vi "maze_v7.vi"   [LabVIEW 2012]
uses:
  <vilib>/NXT/Subs/MotorOutput.ctl
  <vilib>/NXT/Block Support/NXT_InputPort.ctl
  <vilib>/NXT/Dual Mode Library/Motors/MotorBrake.vi
  <vilib>/NXT/Dual Mode Library/Motors/MotorOn.vi
  <vilib>/NXT/Dual Mode Library/Motors/MotorReverse.vi
  <vilib>/NXT/Dual Mode Library/prims/addArrayElements_int.vi
  <vilib>/NXT/Dual Mode Library/Waits/Wait_Num(msec).vi
  <vilib>/NXT/Dual Mode Library/Sound/Tone.vi
types:
  T1 = typedef "MotorOutput.ctl" = u8
  T2 = typedef "LVHSConnector.ctl" = cluster{"Hardware":string, "Flattened String":string}
  T3 = typedef "NXT_InputPort.ctl" = u8
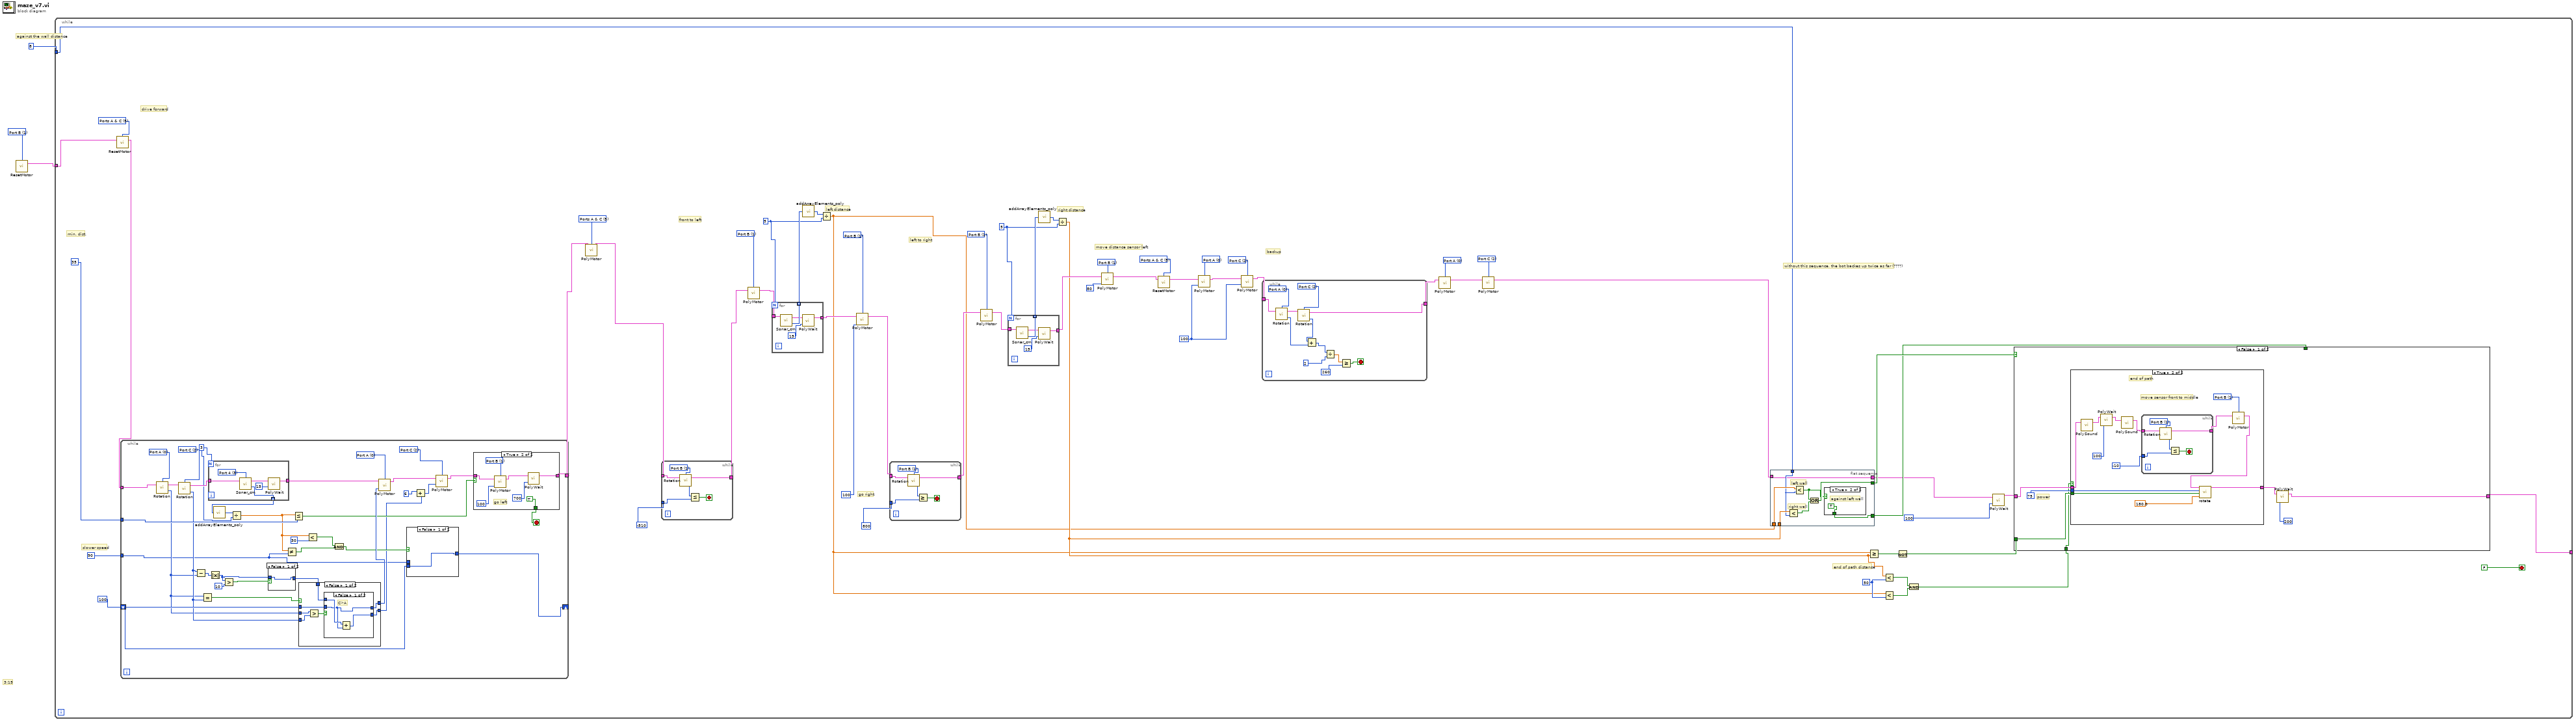
[diagram p0: block diagram]
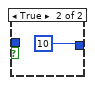
[diagram p2: hidden frame]
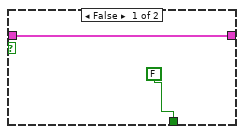
[diagram p4: hidden frame]
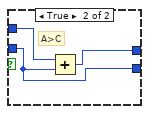
[diagram p5: hidden frame]
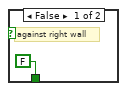
[diagram p7: hidden frame]
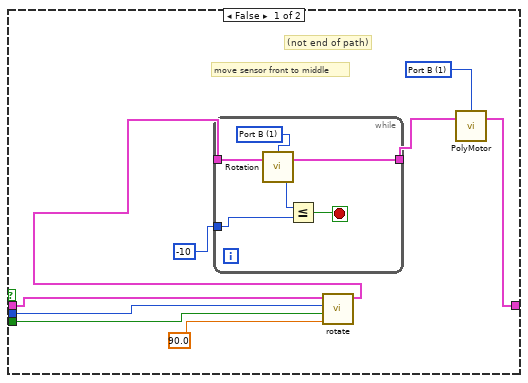
[diagram p8: hidden frame]
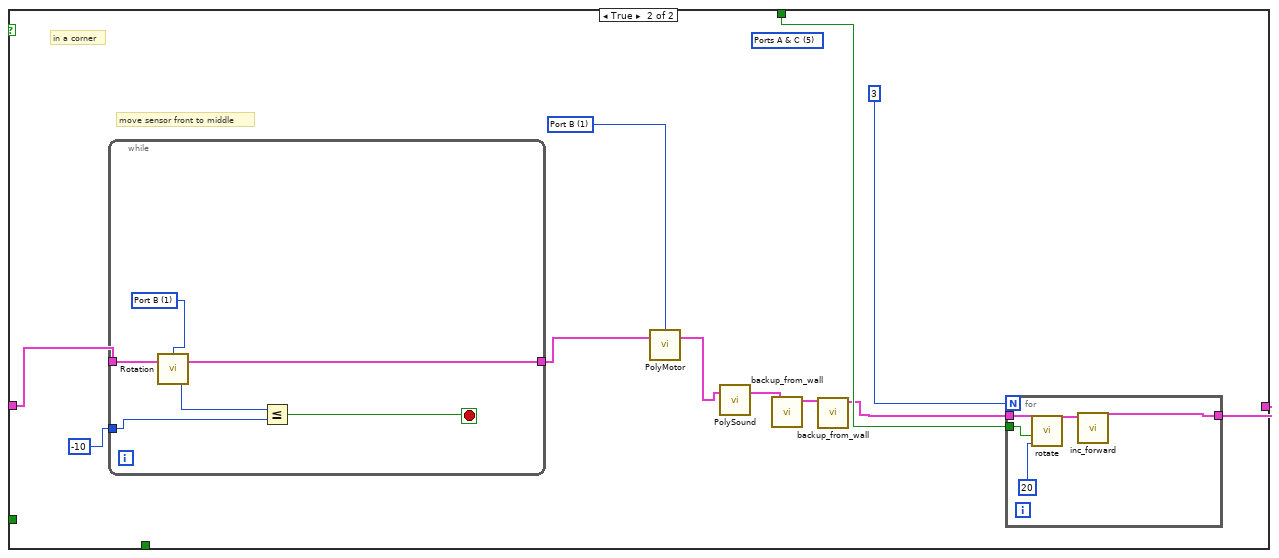
[diagram p9: hidden frame]
diagram:
  w3 = T1 1 items=["Port A"=0, "Port B"=1, "Port C"=2, "Ports A & B"=4, "Ports A & C"=5, "Ports B & C"=6, "All Ports"=3] ("Output Port (All Ports)")
  # "3:15"
  # "against the wall distance"
  n1 = call <vilib>:"ResetMotor.vi"("Port (All Ports)"=w3) -> ("NXT"=w1:T2)  [unwired: 3 in]
  n2 = while {
    tunnel: u16 8 ("power") -> [w57]
    tunnel: [w54] -> _
    tunnel: w1 -> [w46]
    stop <- FALSE stop-if-true
    w7 = u16 50 ("power")
    w14 = T1 1 items=["Port A"=0, "Port B"=1, "Port C"=2, "Ports A & B"=4, "Ports A & C"=5, "Ports B & C"=6, "All Ports"=3] ("Output Port (All Ports)")
    w19 = T1 2 items=["Port A"=0, "Port B"=1, "Port C"=2, "Ports A & B"=4, "Ports A & C"=5, "Ports B & C"=6, "All Ports"=3] ("Output Port (All Ports)")
    w17 = T1 0 items=["Port A"=0, "Port B"=1, "Port C"=2, "Ports A & B"=4, "Ports A & C"=5, "Ports B & C"=6, "All Ports"=3] ("Output Port (All Ports)")
    w21 = 100
    w23 = T1 2 items=["Port A"=0, "Port B"=1, "Port C"=2, "Ports A & B"=4, "Ports A & C"=5, "Ports B & C"=6, "All Ports"=3] ("Output Port (All Ports)")
    w25 = T1 0 items=["Port A"=0, "Port B"=1, "Port C"=2, "Ports A & B"=4, "Ports A & C"=5, "Ports B & C"=6, "All Ports"=3] ("Output Port (All Ports)")
    w26 = T1 5 items=["Port A"=0, "Port B"=1, "Port C"=2, "Ports A & B"=4, "Ports A & C"=5, "Ports B & C"=6, "All Ports"=3] ("Output Port (All Ports)")
    w29 = 5
    w32 = 5
    w39 = T1 1 items=["Port A"=0, "Port B"=1, "Port C"=2, "Ports A & B"=4, "Ports A & C"=5, "Ports B & C"=6, "All Ports"=3] ("Output Port (All Ports)")
    w40 = T1 1 items=["Port A"=0, "Port B"=1, "Port C"=2, "Ports A & B"=4, "Ports A & C"=5, "Ports B & C"=6, "All Ports"=3] ("Output Port (All Ports)")
    w44 = T1 1 items=["Port A"=0, "Port B"=1, "Port C"=2, "Ports A & B"=4, "Ports A & C"=5, "Ports B & C"=6, "All Ports"=3] ("Output Port (All Ports)")
    w53 = T1 5 items=["Port A"=0, "Port B"=1, "Port C"=2, "Ports A & B"=4, "Ports A & C"=5, "Ports B & C"=6, "All Ports"=3] ("Output Port (All Ports)")
    w51 = T1 5 items=["Port A"=0, "Port B"=1, "Port C"=2, "Ports A & B"=4, "Ports A & C"=5, "Ports B & C"=6, "All Ports"=3] ("Output Port (All Ports)")
    # "end of path distance"
    # "move distance sensor left"
    # "backup"
    # "right distance"
    # "left distance"
    # "go right"
    # "left to right"
    # "front to left"
    # "drive forward"
    # "min. dist."
    # "slower speed"
    # "without this sequence, the bot backes up twice as far (????)"
    n3 = call <vilib>:"ResetMotor.vi"("NXT"=w46, "Port (All Ports)"=w51) -> ("NXT"=w52:T2)  [unwired: 2 in]
    n4 = while {
      tunnel: w52 -> [w133]
      tunnel: [w121] -> w50
      tunnel: 35 -> [w123]
      shift-right: [w113] -> _
      shift-left: 100 -> [w112]
      tunnel: 90 -> [w97]
      stop <- w118 stop-if-true
      w98 = 3
      w126 = T1 2 items=["Port A"=0, "Port B"=1, "Port C"=2, "Ports A & B"=4, "Ports A & C"=5, "Ports B & C"=6, "All Ports"=3] ("Output Port (All Ports)")
      w127 = T1 0 items=["Port A"=0, "Port B"=1, "Port C"=2, "Ports A & B"=4, "Ports A & C"=5, "Ports B & C"=6, "All Ports"=3] ("Output Port (All Ports)")
      w128 = T1 2 items=["Port A"=0, "Port B"=1, "Port C"=2, "Ports A & B"=4, "Ports A & C"=5, "Ports B & C"=6, "All Ports"=3] ("Output Port (All Ports)")
      w129 = T1 0 items=["Port A"=0, "Port B"=1, "Port C"=2, "Ports A & B"=4, "Ports A & C"=5, "Ports B & C"=6, "All Ports"=3] ("Output Port (All Ports)")
      n5 = call <vilib>:"Rotation.vi"("NXT"=w133, "Port (Port A)"=w127) -> ("Angle of Rotation"=w110:i32, "NXT"=w132:T2)  [unwired: 1 in]
      n6 = call <vilib>:"Rotation.vi"("NXT"=w132, "Port (Port A)"=w126) -> ("Angle of Rotation"=w111:i32, "NXT"=w131:T2)  [unwired: 1 in]
      n7 = Subtract(x=w111, y=w110) -> (x-y=w109:i32)
      n8 = Equal?(x=w110, y=w111) -> (x = y?=w125:bool)
      n9 = for {
        N: w98 -> [_]
        tunnel: w131 -> [w138]
        tunnel: [w136] -> w124
        tunnel: [w137] -> w101 mode=indexing
        w139 = T3 3 items=["Port 1", "Port 2", "Port 3", "Port 4"] ("Port (Port 4)")
        n10 = call <vilib>:"Sonar_cm.vi"("NXT"=w138, "Port (Port 4)"=w139) -> ("Distance (cm)"=w137:i16, "NXT"=w135:T2)  [unwired: 1 in]
        n11 = call-poly <vilib>:"PolyWait.vi"("Time (100 msec)"=15, "NXT"=w135) -> ("NXT"=w136:T2)  [unwired: 2 in]
      }
      n12 = Absolute Value(x=w109) -> (abs(x)=w106:i32)
      n13 = call-poly <vilib>:"addArrayElements_poly.vi"("Numeric Array"=w101) -> ("Sum"=w100:i32)
      n14 = Greater?(x=w106, y=10) -> (0:w107:bool)
      n15 = Divide(x=w100, y=w98) -> (x/y=w99:dbl)
      n16 = case shown="False" w107 {
        tunnel: [w140 10] -> w105
        tunnel: w106 -> [w140 _]
        frame False {
        }
        frame True {
        }
      }
      n17 = Not Equal?(x=w99, y=w97) -> (x != y?=w115:bool)
      n18 = Less Or Equal?(x=w99, y=w123) -> (x <= y?=w119:bool)
      n19 = case shown="False" w125 {
        tunnel: [w157 w166] -> w122
        tunnel: w112 -> [w158 w166]
        tunnel: [w156 w166] -> w103
        tunnel: w111 -> [w155 _]
        tunnel: w110 -> [w154 _]
        tunnel: w105 -> [w153 _]
        frame False {
          n20 = Greater?(x=w154, y=w155) -> (0:w159:bool)
          n21 = case shown="False" w159 {
            tunnel: w158 -> [w160 w163]
            tunnel: [w160 w165] -> w157
            tunnel: [w162 w163] -> w156
            tunnel: w153 -> [w161 w164]
            frame False {
              # "C>A"
              n22 = Add(x=w161, y=w160) -> (x+y=w162:i32)
            }
            frame True {
              # "A>C"
              n23 = Add(x=w164, y=w163) -> (x+y=w165:i32)
            }
          }
        }
        frame True {
        }
      }
      n24 = Less?(x=w99, y=30) -> (x < y?=w116:bool)
      n25 = And(x=w116, y=w115) -> (x .and. y?=w114:bool)
      n26 = call-poly <vilib>:"PolyMotor.vi"("Power (75)"=w122, "NXT"=w124, "Output Port (All Ports)"=w129) -> ("NXT"=w130:T2)  [unwired: 1 in]
      n27 = case shown="False" w114 {
        tunnel: [w142 w143] -> w113
        tunnel: w112 -> [w142 _]
        tunnel: w97 -> [_ w143]
        frame False {
        }
        frame True {
        }
      }
      n28 = Add(x=6, y=w103) -> (x+y=w102:i32)
      n29 = call-poly <vilib>:"PolyMotor.vi"("Power (75)"=w102, "NXT"=w130, "Output Port (All Ports)"=w128) -> ("NXT"=w120:T2)  [unwired: 1 in]
      n30 = case shown="True" w119 {
        tunnel: [w144 w152] -> w121
        tunnel: w120 -> [w144 w147]
        tunnel: [FALSE TRUE] -> w118
        frame False {
        }
        frame True {
          w149 = T1 1 items=["Port A"=0, "Port B"=1, "Port C"=2, "Ports A & B"=4, "Ports A & C"=5, "Ports B & C"=6, "All Ports"=3] ("Output Port (All Ports)")
          # "go left"
          n31 = call-poly <vilib>:"PolyMotor.vi"("Power (75)"=100, "NXT"=w147, "Output Port (All Ports)"=w149) -> ("NXT"=w146:T2)  [unwired: 1 in]
          n32 = call-poly <vilib>:"PolyWait.vi"("Time (100 msec)"=700, "NXT"=w146) -> ("NXT"=w152:T2)  [unwired: 2 in]
        }
      }
    }
    n33 = call-poly <vilib>:"PolyMotor.vi"("NXT"=w50, "Port (All Ports)"=w53) -> ("NXT"=w27:T2)  [unwired: 2 in]
    n34 = while {
      tunnel: -510 -> [w95]
      tunnel: w27 -> [w93]
      tunnel: [w92] -> w43
      stop <- w91 stop-if-true
      w94 = T1 1 items=["Port A"=0, "Port B"=1, "Port C"=2, "Ports A & B"=4, "Ports A & C"=5, "Ports B & C"=6, "All Ports"=3] ("Output Port (All Ports)")
      n35 = call <vilib>:"Rotation.vi"("NXT"=w93, "Port (Port A)"=w94) -> ("Angle of Rotation"=w96:i32, "NXT"=w92:T2)  [unwired: 1 in]
      n36 = Less Or Equal?(x=w96, y=w95) -> (x <= y?=w91:bool)
    }
    n37 = call-poly <vilib>:"PolyMotor.vi"("NXT"=w43, "Port (All Ports)"=w44) -> ("NXT"=w36:T2)  [unwired: 2 in]
    n38 = for {
      N: w32 -> [_]
      tunnel: w36 -> [w83]
      tunnel: [w84] -> w34 mode=indexing
      tunnel: [w81] -> w35
      n39 = call <vilib>:"Sonar_cm.vi"("NXT"=w83) -> ("Distance (cm)"=w84:i16, "NXT"=w82:T2)  [unwired: 2 in]
      n40 = call-poly <vilib>:"PolyWait.vi"("Time (100 msec)"=15, "NXT"=w82) -> ("NXT"=w81:T2)  [unwired: 2 in]
    }
    n41 = call-poly <vilib>:"addArrayElements_poly.vi"("Numeric Array"=w34) -> ("Sum"=w33:i32)
    n42 = Divide(x=w33, y=w32) -> (x/y=w5:dbl)
    n43 = call-poly <vilib>:"PolyMotor.vi"("Power (75)"=100, "NXT"=w35, "Output Port (All Ports)"=w40) -> ("NXT"=w41:T2)  [unwired: 1 in]
    n44 = while {
      tunnel: 800 -> [w89]
      tunnel: w41 -> [w87]
      tunnel: [w86] -> w38
      stop <- w85 stop-if-true
      w88 = T1 1 items=["Port A"=0, "Port B"=1, "Port C"=2, "Ports A & B"=4, "Ports A & C"=5, "Ports B & C"=6, "All Ports"=3] ("Output Port (All Ports)")
      n45 = call <vilib>:"Rotation.vi"("NXT"=w87, "Port (Port A)"=w88) -> ("Angle of Rotation"=w90:i32, "NXT"=w86:T2)  [unwired: 1 in]
      n46 = Greater Or Equal?(x=w90, y=w89) -> (x >= y?=w85:bool)
    }
    n47 = call-poly <vilib>:"PolyMotor.vi"("NXT"=w38, "Port (All Ports)"=w39) -> ("NXT"=w28:T2)  [unwired: 2 in]
    n48 = for {
      N: w29 -> [_]
      tunnel: w28 -> [w78]
      tunnel: [w79] -> w31 mode=indexing
      tunnel: [w76] -> w13
      n49 = call <vilib>:"Sonar_cm.vi"("NXT"=w78) -> ("Distance (cm)"=w79:i16, "NXT"=w77:T2)  [unwired: 2 in]
      n50 = call-poly <vilib>:"PolyWait.vi"("Time (100 msec)"=15, "NXT"=w77) -> ("NXT"=w76:T2)  [unwired: 2 in]
    }
    n51 = call-poly <vilib>:"addArrayElements_poly.vi"("Numeric Array"=w31) -> ("Sum"=w30:i32)
    n52 = Divide(x=w30, y=w29) -> (x/y=w6:dbl)
    n53 = call-poly <vilib>:"PolyMotor.vi"("Power (75)"=80, "NXT"=w13, "Output Port (All Ports)"=w14) -> ("NXT"=w12:T2)  [unwired: 1 in]
    n54 = call <vilib>:"ResetMotor.vi"("NXT"=w12, "Port (All Ports)"=w26) -> ("NXT"=w20:T2)  [unwired: 2 in]
    n55 = call-poly <vilib>:"PolyMotor.vi"("Power (75)"=w21, "NXT"=w20, "Output Port (All Ports)"=w25) -> ("NXT"=w24:T2)  [unwired: 1 in]
    n56 = call-poly <vilib>:"PolyMotor.vi"("Power (75)"=w21, "NXT"=w24, "Output Port (All Ports)"=w23) -> ("NXT"=w22:T2)  [unwired: 1 in]
    n57 = while {
      tunnel: w22 -> [w72]
      tunnel: [w63] -> w16
      stop <- w65 stop-if-true
      w71 = T1 2 items=["Port A"=0, "Port B"=1, "Port C"=2, "Ports A & B"=4, "Ports A & C"=5, "Ports B & C"=6, "All Ports"=3] ("Output Port (All Ports)")
      w73 = T1 0 items=["Port A"=0, "Port B"=1, "Port C"=2, "Ports A & B"=4, "Ports A & C"=5, "Ports B & C"=6, "All Ports"=3] ("Output Port (All Ports)")
      n58 = call <vilib>:"Rotation.vi"("NXT"=w72, "Port (Port A)"=w73) -> ("Angle of Rotation"=w68:i32, "NXT"=w74:T2)  [unwired: 1 in]
      n59 = call <vilib>:"Rotation.vi"("NXT"=w74, "Port (Port A)"=w71) -> ("Angle of Rotation"=w67:i32, "NXT"=w63:T2)  [unwired: 1 in]
      n60 = Add(x=w67, y=w68) -> (x+y=w69:i32)
      n61 = Divide(x=w69, y=2) -> (x/y=w64:dbl)
      n62 = Greater Or Equal?(x=w64, y=260) -> (x >= y?=w65:bool)
    }
    n63 = call-poly <vilib>:"PolyMotor.vi"("NXT"=w16, "Port (All Ports)"=w17) -> ("NXT"=w18:T2)  [unwired: 2 in]
    n64 = call-poly <vilib>:"PolyMotor.vi"("NXT"=w18, "Port (All Ports)"=w19) -> ("NXT"=w11:T2)  [unwired: 2 in]
    n65 = flat-sequence {
      tunnel: [w167] -> w10
      tunnel: w6 -> [w174]
      tunnel: w57 -> [w172]
      tunnel: w5 -> [w173]
      tunnel: [w170] -> w56
      tunnel: [w168] -> w55
      tunnel: w11 -> [w167]
      frame #0 {
        # "left wall"
        # "right wall"
        n66 = Less?(x=w174, y=w172) -> (x < y?=w171:bool)
        n67 = Less?(x=w173, y=w172) -> (x < y?=w169:bool)
        n68 = Or(x=w169, y=w171) -> (x .or. y?=w170:bool)
        n69 = case shown="True" w169 {
          tunnel: [FALSE TRUE] -> w168
          frame False {
            # "against right wall"
          }
          frame True {
            # "against left wall"
          }
        }
      }
    }
    n70 = Greater Or Equal?(x=w5, y=w6) -> (x >= y?=w61:bool)
    n71 = Less?(x=w6, y=w7) -> (x < y?=w9:bool)
    n72 = Less?(x=w5, y=w7) -> (x < y?=w8:bool)
    n73 = Not(x=w61) -> (.not. x?=w60:bool)
    n74 = And(x=w9, y=w8) -> (x .and. y?=w4:bool)
    n75 = call-poly <vilib>:"PolyWait.vi"("Time (100 msec)"=u16 100 ("power"), "NXT"=w10) -> ("NXT"=w59:T2)  [unwired: 2 in]
    n76 = case shown="False" w56 {
      tunnel: w55 -> [_ w225]
      tunnel: w59 -> [w180 w219]
      tunnel: [w179 w223] -> w54
      tunnel: w60 -> [w182 _]
      tunnel: w4 -> [w178 _]
      frame False {
        # "power"
        n77 = case shown="True" w178 {
          tunnel: u16 75 ("power") -> [w190 w211]
          tunnel: w182 -> [w189 w210]
          tunnel: w180 -> [w191 w199]
          tunnel: [w184 w208] -> w177
          frame False {
            w187 = T1 1 items=["Port A"=0, "Port B"=1, "Port C"=2, "Ports A & B"=4, "Ports A & C"=5, "Ports B & C"=6, "All Ports"=3] ("Output Port (All Ports)")
            # "move sensor front to middle"
            # "(not end of path)"
            n78 = call "rotate.vi"("degrees to  rotate"=90.0, "right(T)/left(F)"=w189, "power"=w190, "NXT 2"=w191) -> ("NXT"=w185:T2)  [unwired: 7 in]
            n79 = while {
              tunnel: -10 -> [w197]
              tunnel: [w195] -> w186
              tunnel: w185 -> [w193]
              stop <- w194 stop-if-true
              w196 = T1 1 items=["Port A"=0, "Port B"=1, "Port C"=2, "Ports A & B"=4, "Ports A & C"=5, "Ports B & C"=6, "All Ports"=3] ("Output Port (All Ports)")
              n80 = call <vilib>:"Rotation.vi"("NXT"=w193, "Port (Port A)"=w196) -> ("Angle of Rotation"=w198:i32, "NXT"=w195:T2)  [unwired: 1 in]
              n81 = Less Or Equal?(x=w198, y=w197) -> (x <= y?=w194:bool)
            }
            n82 = call-poly <vilib>:"PolyMotor.vi"("NXT"=w186, "Port (All Ports)"=w187) -> ("NXT"=w184:T2)  [unwired: 2 in]
          }
          frame True {
            w206 = T1 1 items=["Port A"=0, "Port B"=1, "Port C"=2, "Ports A & B"=4, "Ports A & C"=5, "Ports B & C"=6, "All Ports"=3] ("Output Port (All Ports)")
            # "move sensor front to middle"
            # "end of path"
            n83 = call-poly <vilib>:"PolySound.vi"("NXT"=w199) -> ("NXT"=w202:T2)  [unwired: 3 in]
            n84 = call-poly <vilib>:"PolyWait.vi"("Time (100 msec)"=100, "NXT"=w202) -> ("NXT"=w201:T2)  [unwired: 2 in]
            n85 = call-poly <vilib>:"PolySound.vi"("NXT"=w201) -> ("NXT"=w200:T2)  [unwired: 3 in]
            n86 = while {
              tunnel: -10 -> [w216]
              tunnel: [w214] -> w205
              tunnel: w200 -> [w212]
              stop <- w213 stop-if-true
              w215 = T1 1 items=["Port A"=0, "Port B"=1, "Port C"=2, "Ports A & B"=4, "Ports A & C"=5, "Ports B & C"=6, "All Ports"=3] ("Output Port (All Ports)")
              n87 = call <vilib>:"Rotation.vi"("NXT"=w212, "Port (Port A)"=w215) -> ("Angle of Rotation"=w217:i32, "NXT"=w214:T2)  [unwired: 1 in]
              n88 = Less Or Equal?(x=w217, y=w216) -> (x <= y?=w213:bool)
            }
            n89 = call-poly <vilib>:"PolyMotor.vi"("NXT"=w205, "Port (All Ports)"=w206) -> ("NXT"=w204:T2)  [unwired: 2 in]
            n90 = call "rotate.vi"("degrees to  rotate"=180.0, "right(T)/left(F)"=w210, "power"=w211, "NXT 2"=w204) -> ("NXT"=w208:T2)  [unwired: 7 in]
          }
        }
        n91 = call-poly <vilib>:"PolyWait.vi"("Time (100 msec)"=i16 200 ("degrees to  rotate"), "NXT"=w177) -> ("NXT"=w179:T2)  [unwired: 2 in]
      }
      frame True {
        w221 = T1 1 items=["Port A"=0, "Port B"=1, "Port C"=2, "Ports A & B"=4, "Ports A & C"=5, "Ports B & C"=6, "All Ports"=3] ("Output Port (All Ports)")
        (unwired) T1 5 items=["Port A"=0, "Port B"=1, "Port C"=2, "Ports A & B"=4, "Ports A & C"=5, "Ports B & C"=6, "All Ports"=3] ("Output Port (All Ports)")
        # "move sensor front to middle"
        # "in a corner"
        n92 = while {
          tunnel: -10 -> [w233]
          tunnel: [w231] -> w220
          tunnel: w219 -> [w229]
          stop <- w230 stop-if-true
          w232 = T1 1 items=["Port A"=0, "Port B"=1, "Port C"=2, "Ports A & B"=4, "Ports A & C"=5, "Ports B & C"=6, "All Ports"=3] ("Output Port (All Ports)")
          n93 = call <vilib>:"Rotation.vi"("NXT"=w229, "Port (Port A)"=w232) -> ("Angle of Rotation"=w234:i32, "NXT"=w231:T2)  [unwired: 1 in]
          n94 = Less Or Equal?(x=w234, y=w233) -> (x <= y?=w230:bool)
        }
        n95 = call-poly <vilib>:"PolyMotor.vi"("NXT"=w220, "Port (All Ports)"=w221) -> ("NXT"=w218:T2)  [unwired: 2 in]
        n96 = call-poly <vilib>:"PolySound.vi"("NXT"=w218) -> ("NXT"=w228:T2)  [unwired: 3 in]
        n97 = call "backup_from_wall.vi"("NXT"=w228) -> ("NXT2"=w227:T2)  [unwired: 10 in]
        n98 = call "backup_from_wall.vi"("NXT"=w227) -> ("NXT2"=w224:T2)  [unwired: 10 in]
        n99 = for {
          N: u16 3 ("power") -> [_]
          tunnel: w225 -> [w238]
          tunnel: w224 -> [w237]
          tunnel: [w235] -> w223
          n100 = call "rotate.vi"("degrees to  rotate"=u16 20 ("power"), "right(T)/left(F)"=w238, "NXT 2"=w237) -> ("NXT"=w236:T2)  [unwired: 8 in]
          n101 = call "inc_forward.vi"("NXT"=w236) -> ("NXT2"=w235:T2)  [unwired: 10 in]
        }
      }
    }
  }
